vi "Acquisition next state logic.vi"(0 "Message Queues":T5, 5 "Acquired z-plane index":i32, 7 "Logging queue element":T1={"Imaging Protocol"=enum."Live Imaging", "Number of Trials"=0, "Frame Size"=512, "# Averaged frames"=0, "Dwell time (us)"=0.0, "Index of Z-plane"=0, "Timelapse?"=FALSE, "Logging process is active"=FALSE, "Speed logging enabled"=FALSE, "tdms file ref"=refnum, "path"=path "", "Trial Number"=0, "Expected # points acquired"=FALSE, "Manually stopped"=FALSE, "Ch0 data"=[], "Ch1 data"=[], "Last trial"=FALSE, "Points acquired"={"Ch0 last trial"=0, "Ch1 last trial"=0, "All trials"=0}} {"Frame Size" items=["100X100"=100, "128X128"=128, "200X200"=200, "256X256"=256, "512X512"=512, "1024x1024"=1024, "2048x2048"=2048]; "Dwell time (us)" format="%#.6g"}, 9 "Imaging Protocol":T2=enum."Live Imaging", 11 "error in":errorcluster) -> (6 "Index of next Z-plane to acquire":i32, 15 "error out":errorcluster)   [LabVIEW 2013]
uses:
  User Interface/Queue/Message Queue/Typedefs/All Message Queues.ctl
  User Interface/Queue/Message Queue/Typedefs/Message Cluster.ctl
  Typedefs/Logging queue element.ctl
  Typedefs/Imaging Protocols enum.ctl
  Typedefs/Frame Size.ctl
  Typedefs/Acquired points count.ctl
  Typedefs/Read Write Enum.ctl
  Global Variables/General Globals.vi
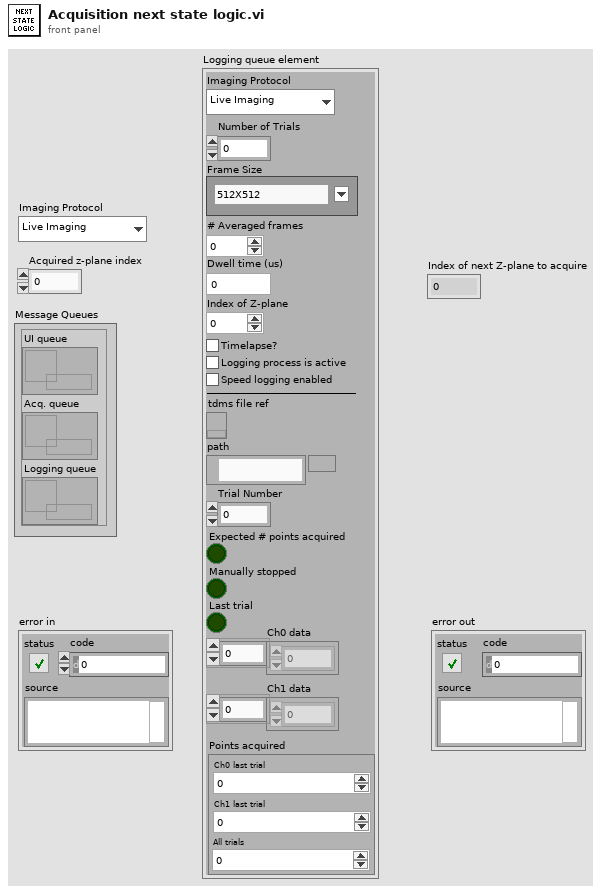
[diagram p1: front panel]
types:
  T1 = typedef "Logging queue element.ctl" = cluster{"Imaging Protocol":T2, "Number of Trials":u16, "Frame Size":T3, "# Averaged frames":u16, "Dwell time (us)":dbl, "Index of Z-plane":i32, "Timelapse?":bool, "Logging process is active":bool, "Speed logging enabled":bool, "tdms file ref":refnum<k34>, "path":path, "Trial Number":i32, "Expected # points acquired":bool, "Manually stopped":bool, "Ch0 data":u32[], "Ch1 data":u32[], "Last trial":bool, "Points acquired":T4}
  T2 = typedef "Imaging Protocols enum.ctl" = enum16{"AOL Z-Stack", "Motor Z Stack", "Functional Acquisition", "Single Plane Acquisition", "Volume Acquisition", "Live Imaging", "Live Plane Imaging", "Live Volume Imaging"}
  T3 = typedef "Frame Size.ctl" = u16
  T4 = typedef "Acquired points count.ctl" = cluster{"Ch0 last trial":u64, "Ch1 last trial":u64, "All trials":u64}
  T5 = typedef "All Message Queues.ctl" = cluster{"UI queue":refnum<queue>, "Acq. queue":refnum<queue>, "Logging queue":refnum<queue>}
  T6 = typedef "Read Write Enum.ctl" = enum16{"Read", "Write"}
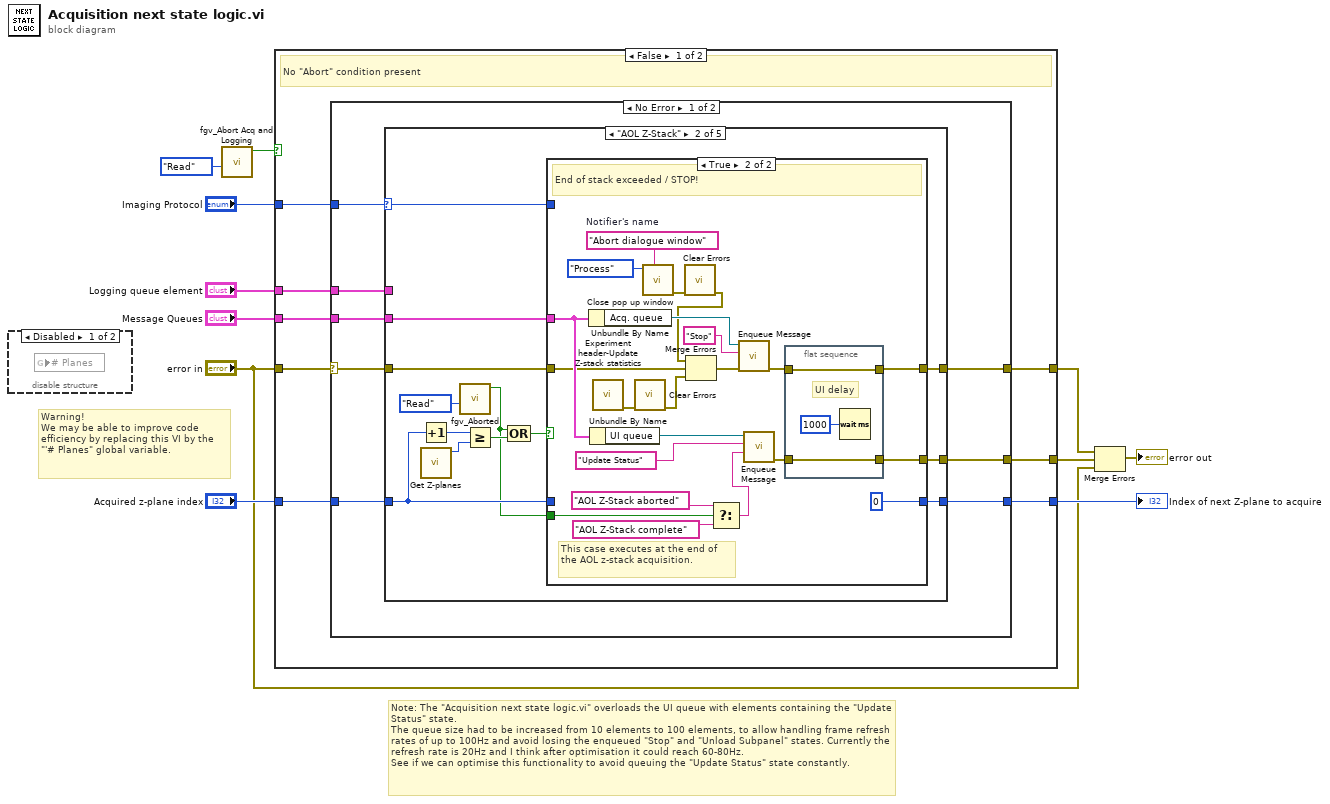
[diagram p0: block diagram]
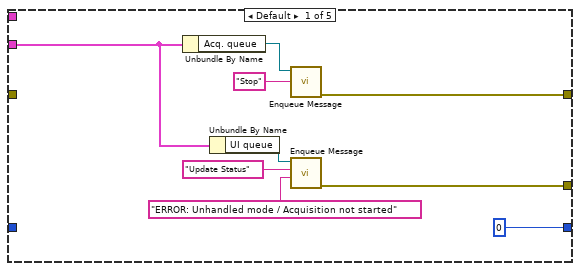
[diagram p3: hidden frame]
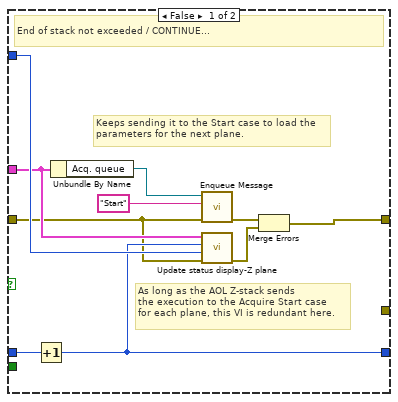
[diagram p4: hidden frame]
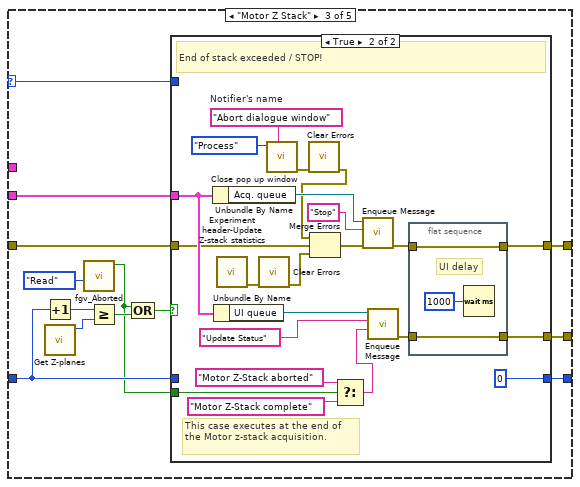
[diagram p5: hidden frame]
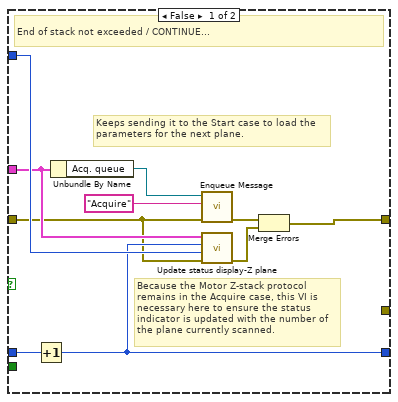
[diagram p6: hidden frame]
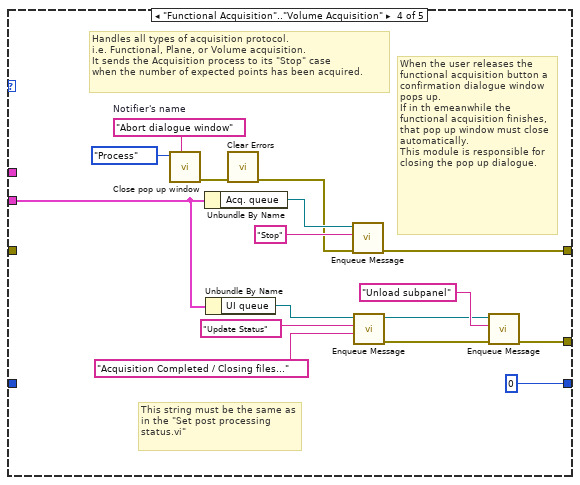
[diagram p7: hidden frame]
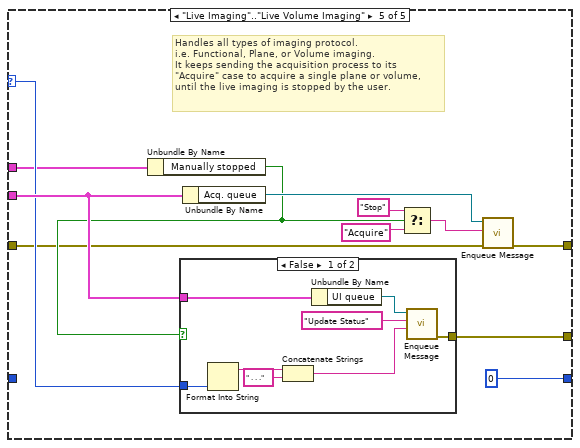
[diagram p8: hidden frame]
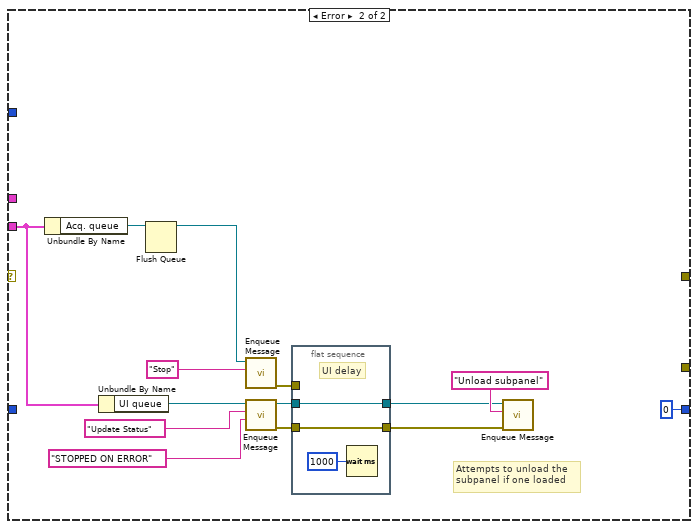
[diagram p10: hidden frame]
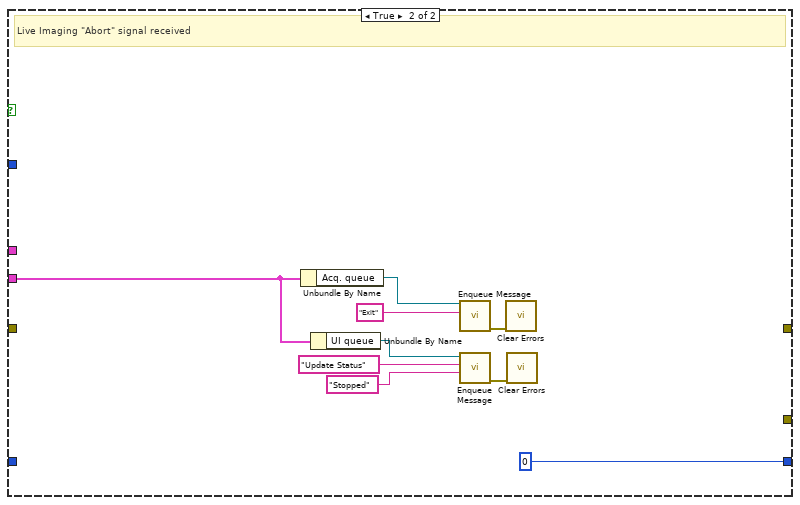
[diagram p11: hidden frame]
diagram:
  # "Note: The \"Acquisition next state logic.vi\" overloads the UI queue with elements containing the \"Update Status\" state.\nThe queue size had to be increased from 10 elements to 100 elements, to allow handling frame refresh rates of up to 100Hz and avoid losing the enqueued \"Stop\" and \"Unload Subpanel\" states. Currently the refresh rate is 20Hz and I think after optimisation it could reach 60-80Hz.\nSee if we can optimise this functionality to avoid queuing the \"Update Status\" state constantly."
  # "Warning!\nWe may be able to improve code efficiency by replacing this VI by the \"'# Planes\" global variable."
  n1 = disable-structure "Diagram Disable Structure" shown="Disabled" {
    frame Disabled {
      n2 = global read "General Globals.vi" "# Planes"() -> ()  [unwired: 1 in]
    }
    frame Enabled {
    }
  }
  n3 = call "fgv_Abort Acq and Logging.vi"("Function"=Read_Write_Enum."Read") -> ("Abort acquisition"=w1:bool)  [unwired: 9 in, 1 out]
  n4 = case shown="False" w1 {
    tunnel: [w19 _] -> w7
    tunnel: "error in" -> [w12 _]
    tunnel: [w18 0] -> w8
    tunnel: [w17 _] -> w6
    tunnel: "Acquired z-plane index" -> [w16 _]
    tunnel: "Imaging Protocol" -> [w14 _]
    tunnel: "Message Queues" -> [w15 w188]
    tunnel: "Logging queue element" -> [w13 _]
    frame False {
      # "No \"Abort\" condition present"
      n5 = case shown="No Error" w12 {
        selector: w12 -> [w20 _]
        tunnel: [w27 _] -> w19
        tunnel: [w26 0] -> w18
        tunnel: [w25 _] -> w17
        tunnel: w16 -> [w24 _]
        tunnel: w15 -> [w23 w173]
        tunnel: w14 -> [w22 _]
        tunnel: w13 -> [w21 _]
        frame No Error {
          n6 = case shown="\"AOL Z-Stack\"" w22 {
            selector: w22 -> [_ w41 w89 _ w157]
            tunnel: w20 -> [_ w44 w92 _ w150]
            tunnel: [w35 w48 w96 w147 w160] -> w27
            tunnel: [0 w46 w94 0 0] -> w26
            tunnel: w24 -> [_ w45 w93 _ _]
            tunnel: [w32 w47 w95 w139 w149] -> w25
            tunnel: w23 -> [w29 w43 w91 w143 w158]
            tunnel: w21 -> [_ _ _ _ w156]
            frame Default {
              n7 = Unbundle By Name(w29) -> ("Acq. queue"=w30:refnum<queue>)
              n8 = Unbundle By Name(w29) -> ("UI queue"=w31:refnum<queue>)
              n9 = call "Enqueue Message.vi"("Message"="Stop", "Queue"=w30) -> ("error out"=w35:errorcluster)  [unwired: 8 in, 1 out]
              n10 = call "Enqueue Message.vi"("Message Data"="ERROR: Unhandled mode / Acquisition not started" ("Message"), "Message"="Update Status", "Queue"=w31) -> ("error out"=w32:errorcluster)  [unwired: 7 in, 1 out]
            }
            frame "AOL Z-Stack" {
              n11 = Increment(x=w45) -> (x+1=w42:i32)
              n12 = call "Get Z-planes.vi"() -> ("# of Z-planes"=w49:i32)  [unwired: 7 in, 4 out]
              n13 = call "fgv_Aborted.vi"("Function"=Read_Write_Enum."Read") -> ("Funct Acq Aborted?"=w37:bool)  [unwired: 9 in, 1 out]
              n14 = Greater Or Equal?(x=w42, y=w49) -> (x >= y?=w39:bool)
              n15 = Compound Arithmetic op=OR(w37, w39) -> (w38:bool)
              n16 = case shown="True" w38 {
                tunnel: [w50 w74] -> w48
                tunnel: w44 -> [w53 w68]
                tunnel: w45 -> [w58 _]
                tunnel: [w54 0] -> w46
                tunnel: [_ w72] -> w47
                tunnel: w43 -> [w55 w78]
                tunnel: w41 -> [w56 _]
                tunnel: w37 -> [_ w60]
                frame False {
                  # "As long as the AOL Z-stack sends\nthe execution to the Acquire Start case\nfor each plane, this VI is redundant here."
                  # "Keeps sending it to the Start case to load the\nparameters for the next plane."
                  # "End of stack not exceeded / CONTINUE..."
                  n17 = Increment(x=w58) -> (x+1=w54:i32)
                  n18 = Unbundle By Name(w55) -> ("Acq. queue"=w57:refnum<queue>)
                  n19 = call "Enqueue Message.vi"("error in (no error)"=w53, "Message"="Start", "Queue"=w57) -> ("error out"=w51:errorcluster)  [unwired: 7 in, 1 out]
                  n20 = call "Update status display-Z plane.vi"("error in (no error)"=w53, "Imaging Protocol"=w56, "Acquired z-plane index"=w54, "Message Queues"=w55) -> ("error out"=w52:errorcluster)  [unwired: 7 in]
                  n21 = Merge Errors(w51, w52) -> (w50:errorcluster)
                }
                frame True {
                  w66 = "Abort dialogue window"  # Notifier's name
                  # "This case executes at the end of the AOL z-stack acquisition."
                  # "End of stack exceeded / STOP!"
                  n22 = Unbundle By Name(w78) -> ("Acq. queue"=w79:refnum<queue>)
                  n23 = Unbundle By Name(w78) -> ("UI queue"=w77:refnum<queue>)
                  n24 = call "Experiment header-Update Z-stack statistics.vi"() -> ("error out"=w71:errorcluster)  [unwired: 11 in]
                  n25 = call <vilib>:"Clear Errors.vi"("error in (no error)"=w71) -> ("error out"=w70:errorcluster)  [unwired: 6 in]
                  n26 = call "Close pop up window.vi"("Notifier's name"=w66, "Location"=enum16{"Window", "Process"}."Process") -> ("error out"=w65:errorcluster)  [unwired: 7 in, 2 out]
                  n27 = call <vilib>:"Clear Errors.vi"("error in (no error)"=w65) -> ("error out"=w64:errorcluster)  [unwired: 6 in]
                  n28 = Merge Errors(w64, w68, w70) -> (w69:errorcluster)
                  n29 = Select(t="AOL Z-Stack aborted" ("Message"), s=w60, f="AOL Z-Stack complete" ("Message")) -> (s? t:f=w62:string)
                  n30 = call "Enqueue Message.vi"("error in (no error)"=w69, "Message"="Stop", "Queue"=w79) -> ("error out"=w75:errorcluster)  [unwired: 7 in, 1 out]
                  n31 = call "Enqueue Message.vi"("Message Data"=w62, "Message"="Update Status", "Queue"=w77) -> ("error out"=w73:errorcluster)  [unwired: 7 in, 1 out]
                  n32 = flat-sequence {
                    tunnel: w75 -> [w83]
                    tunnel: [w83] -> w74
                    tunnel: w73 -> [w82]
                    tunnel: [w82] -> w72
                    frame #0 {
                      # "UI delay"
                      n33 = Wait (ms)(milliseconds to wait=u32 1000) -> ()  [unwired: 1 out]
                    }
                  }
                }
              }
            }
            frame "Motor Z Stack" {
              n34 = Increment(x=w93) -> (x+1=w90:i32)
              n35 = call "Get Z-planes.vi"() -> ("# of Z-planes"=w97:i32)  [unwired: 7 in, 4 out]
              n36 = call "fgv_Aborted.vi"("Function"=Read_Write_Enum."Read") -> ("Funct Acq Aborted?"=w85:bool)  [unwired: 9 in, 1 out]
              n37 = Greater Or Equal?(x=w90, y=w97) -> (x >= y?=w87:bool)
              n38 = Compound Arithmetic op=OR(w85, w87) -> (w86:bool)
              n39 = case shown="True" w86 {
                tunnel: [w98 w122] -> w96
                tunnel: w92 -> [w101 w116]
                tunnel: w93 -> [w106 _]
                tunnel: [w102 0] -> w94
                tunnel: [_ w120] -> w95
                tunnel: w91 -> [w103 w126]
                tunnel: w89 -> [w104 _]
                tunnel: w85 -> [_ w108]
                frame False {
                  # "Because the Motor Z-stack protocol\nremains in the Acquire case, this VI is necessary here to ensure the status indicator is updated with the number of the plane currently scanned."
                  # "Keeps sending it to the Start case to load the\nparameters for the next plane."
                  # "End of stack not exceeded / CONTINUE..."
                  n40 = Increment(x=w106) -> (x+1=w102:i32)
                  n41 = Unbundle By Name(w103) -> ("Acq. queue"=w105:refnum<queue>)
                  n42 = call "Enqueue Message.vi"("error in (no error)"=w101, "Message"="Acquire", "Queue"=w105) -> ("error out"=w99:errorcluster)  [unwired: 7 in, 1 out]
                  n43 = call "Update status display-Z plane.vi"("error in (no error)"=w101, "Imaging Protocol"=w104, "Acquired z-plane index"=w102, "Message Queues"=w103) -> ("error out"=w100:errorcluster)  [unwired: 7 in]
                  n44 = Merge Errors(w99, w100) -> (w98:errorcluster)
                }
                frame True {
                  w114 = "Abort dialogue window"  # Notifier's name
                  # "This case executes at the end of the Motor z-stack acquisition."
                  # "End of stack exceeded / STOP!"
                  n45 = Unbundle By Name(w126) -> ("Acq. queue"=w127:refnum<queue>)
                  n46 = Unbundle By Name(w126) -> ("UI queue"=w125:refnum<queue>)
                  n47 = call "Experiment header-Update Z-stack statistics.vi"() -> ("error out"=w119:errorcluster)  [unwired: 11 in]
                  n48 = call <vilib>:"Clear Errors.vi"("error in (no error)"=w119) -> ("error out"=w118:errorcluster)  [unwired: 6 in]
                  n49 = call "Close pop up window.vi"("Notifier's name"=w114, "Location"=enum16{"Window", "Process"}."Process") -> ("error out"=w113:errorcluster)  [unwired: 7 in, 2 out]
                  n50 = call <vilib>:"Clear Errors.vi"("error in (no error)"=w113) -> ("error out"=w112:errorcluster)  [unwired: 6 in]
                  n51 = Merge Errors(w112, w116, w118) -> (w117:errorcluster)
                  n52 = Select(t="Motor Z-Stack aborted" ("Message"), s=w108, f="Motor Z-Stack complete" ("Message")) -> (s? t:f=w110:string)
                  n53 = call "Enqueue Message.vi"("error in (no error)"=w117, "Message"="Stop", "Queue"=w127) -> ("error out"=w123:errorcluster)  [unwired: 7 in, 1 out]
                  n54 = call "Enqueue Message.vi"("Message Data"=w110, "Message"="Update Status", "Queue"=w125) -> ("error out"=w121:errorcluster)  [unwired: 7 in, 1 out]
                  n55 = flat-sequence {
                    tunnel: w123 -> [w131]
                    tunnel: [w131] -> w122
                    tunnel: w121 -> [w130]
                    tunnel: [w130] -> w120
                    frame #0 {
                      # "UI delay"
                      n56 = Wait (ms)(milliseconds to wait=u32 1000) -> ()  [unwired: 1 out]
                    }
                  }
                }
              }
            }
            frame "Functional Acquisition".."Volume Acquisition" {
              w136 = "Abort dialogue window"  # Notifier's name
              # "When the user releases the functional acquisition button a confirmation dialogue window pops up.\nIf in th emeanwhile the functional acquisition finishes, that pop up window must close automatically.\nThis module is responsible for closing the pop up dialogue."
              # "This string must be the same as in the \"Set post processing status.vi\""
              # "Handles all types of acquisition protocol.\ni.e. Functional, Plane, or Volume acquisition.\nIt sends the Acquisition process to its \"Stop\" case\nwhen the number of expected points has been acquired."
              n57 = call "Close pop up window.vi"("Notifier's name"=w136, "Location"=enum16{"Window", "Process"}."Process") -> ("error out"=w134:errorcluster)  [unwired: 7 in, 2 out]
              n58 = Unbundle By Name(w143) -> ("Acq. queue"=w144:refnum<queue>)
              n59 = Unbundle By Name(w143) -> ("UI queue"=w142:refnum<queue>)
              n60 = call <vilib>:"Clear Errors.vi"("error in (no error)"=w134) -> ("error out"=w133:errorcluster)  [unwired: 6 in]
              n61 = call "Enqueue Message.vi"("error in (no error)"=w133, "Message"="Stop", "Queue"=w144) -> ("error out"=w147:errorcluster)  [unwired: 7 in, 1 out]
              n62 = call "Enqueue Message.vi"("Message Data"="Acquisition Completed / Closing files..." ("Message"), "Message"="Update Status", "Queue"=w142) -> ("error out"=w140:errorcluster, "Queue out"=w138:refnum<queue>)  [unwired: 7 in]
              n63 = call "Enqueue Message.vi"("error in (no error)"=w140, "Message"="Unload subpanel", "Queue"=w138) -> ("error out"=w139:errorcluster)  [unwired: 7 in, 1 out]
            }
            frame "Live Imaging".."Live Volume Imaging" {
              # "Handles all types of imaging protocol.\ni.e. Functional, Plane, or Volume imaging.\nIt keeps sending the acquisition process to its\n\"Acquire\" case to acquire a single plane or volume,\nuntil the live imaging is stopped by the user."
              n64 = Unbundle By Name(w156) -> ("Manually stopped"=w151:bool)
              n65 = case shown="False" w151 {
                tunnel: w158 -> [w166 _]
                tunnel: w157 -> [w165 _]
                tunnel: [w162 _] -> w149
                frame False {
                  n66 = Format Into String(w165) -> (resulting string=w164:string)  [unwired: 3 in, 1 out]
                  n67 = Concatenate Strings(w164, " . . ." ("string")) -> (w161:string)
                  n68 = Unbundle By Name(w166) -> ("UI queue"=w167:refnum<queue>)
                  n69 = call "Enqueue Message.vi"("Message Data"=w161, "Message"="Update Status", "Queue"=w167) -> ("error out"=w162:errorcluster)  [unwired: 7 in, 1 out]
                }
                frame True {
                }
              }
              n70 = Unbundle By Name(w158) -> ("Acq. queue"=w159:refnum<queue>)
              n71 = Select(t="Stop" ("Message"), s=w151, f="Acquire" ("Message")) -> (s? t:f=w153:string)
              n72 = call "Enqueue Message.vi"("error in (no error)"=w150, "Message"=w153, "Queue"=w159) -> ("error out"=w160:errorcluster)  [unwired: 7 in, 1 out]
            }
          }
        }
        frame Error {
          # "Attempts to unload the\nsubpanel if one loaded"
          n73 = Unbundle By Name(w173) -> ("Acq. queue"=w182:refnum<queue>)
          n74 = Unbundle By Name(w173) -> ("UI queue"=w176:refnum<queue>)
          n75 = Flush Queue(queue=w182) -> (queue out=w174:refnum<queue>)  [unwired: 1 in, 2 out]
          n76 = call "Enqueue Message.vi"("Message"="Stop", "Queue"=w174) -> ("error out"=w179:errorcluster)  [unwired: 8 in, 1 out]
          n77 = call "Enqueue Message.vi"("Message Data"="STOPPED ON ERROR" ("Message"), "Message"="Update Status", "Queue"=w176) -> ("error out"=w180:errorcluster, "Queue out"=w170:refnum<queue>)  [unwired: 7 in]
          n78 = flat-sequence {
            tunnel: w179 -> [_]
            tunnel: w180 -> [w184]
            tunnel: [w184] -> w171
            tunnel: [w183] -> w169
            tunnel: w170 -> [w183]
            frame #0 {
              # "UI delay"
              n79 = Wait (ms)(milliseconds to wait=u32 1000) -> ()  [unwired: 1 out]
            }
          }
          n80 = call "Enqueue Message.vi"("error in (no error)"=w171, "Message"="Unload subpanel", "Queue"=w169) -> ()  [unwired: 7 in, 2 out]
        }
      }
    }
    frame True {
      # "Live Imaging \"Abort\" signal received"
      n81 = Unbundle By Name(w188) -> ("Acq. queue"=w192:refnum<queue>)
      n82 = Unbundle By Name(w188) -> ("UI queue"=w189:refnum<queue>)
      n83 = call "Enqueue Message.vi"("Message"="Exit", "Queue"=w192) -> ("error out"=w186:errorcluster)  [unwired: 8 in, 1 out]
      n84 = call "Enqueue Message.vi"("Message Data"="Stopped" ("Message"), "Message"="Update Status", "Queue"=w189) -> ("error out"=w187:errorcluster)  [unwired: 7 in, 1 out]
      n85 = call <vilib>:"Clear Errors.vi"("error in (no error)"=w186) -> ()  [unwired: 6 in, 1 out]
      n86 = call <vilib>:"Clear Errors.vi"("error in (no error)"=w187) -> ()  [unwired: 6 in, 1 out]
    }
  }
  "Index of next Z-plane to acquire" <- w8
  n87 = Merge Errors(w7, w6, "error in") -> (→"error out":errorcluster)
